vi "Exit.vi"(8 "error in (no error)":errorcluster, 11 "Running in":refnum<class "Running.lvclass">) -> (0 "error out":errorcluster, 3 "Running out":refnum<class "Running.lvclass">)   [LabVIEW 2013, in "Process States.lvlib" / "Running.lvclass"]
doc: "This override sends a Stop Acquisition message to the Process Actor. It also sends a Log Event message to the UI, with the string containing \"Exiting Running State\", the average value of the data stream, and the total number of elements of the steam as its payload."
uses:
  Running.lvclass
  <vilib>/ActorFramework/Actor/Actor.lvclass/Actor.ctl
  Process State/Process State.lvclass
  Process State/Process State.lvclass/Process State.ctl
  Running.lvclass/Running.ctl
  State Pattern UI/Log Event Msg/Log Event Msg.lvclass/Log Event Msg.ctl
  <vilib>/ActorFramework/Message Enqueuer/Message Enqueuer.lvclass/Message Enqueuer.ctl
  <vilib>/ActorFramework/Message Enqueuer/Enqueue.vi
  <vilib>/ActorFramework/Message Priority Queue/Priority Enqueue.vi
  State Pattern UI/Log Event Msg/Log Event Msg.lvclass
  Process Actor/Process Messages/Stop Acquisition Msg/Stop Acquisition Msg.lvclass
  <vilib>/ActorFramework/Actor/Actor.lvclass
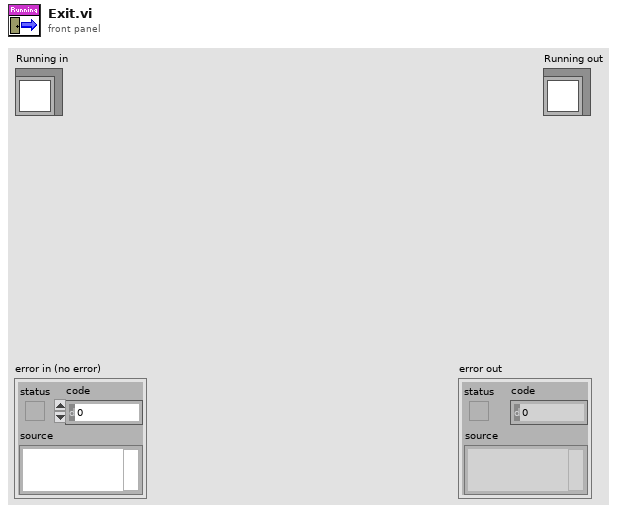
[diagram p1: front panel]
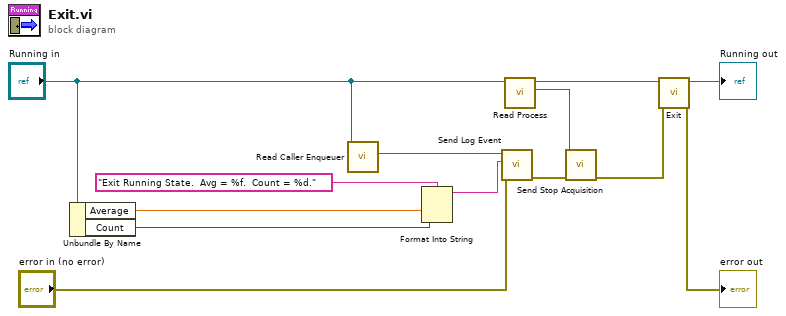
[diagram p0: block diagram]
diagram:
  n1 = Unbundle By Name("Running in") -> ("Average"=w13:dbl, "Count"=w10:i32)
  n2 = call <vilib>:"Read Caller Enqueuer.vi"("Actor"="Running in") -> ("Caller Enqueuer"=w9:refnum<class "Message Enqueuer.lvclass">)  [unwired: 10 in]
  n3 = Format Into String(format string="Exit Running State.  Avg = %f.  Count = %d." ("Event Text"), w13, w10) -> (resulting string=w11:string)  [unwired: 2 in, 1 out]
  n4 = call "Send Log Event.vi"("error in (no error)"="error in (no error)", "Event Text"=w11, "Message Enqueuer"=w9) -> ("error out"=w4:errorcluster)  [unwired: 8 in]
  n5 = call "Read Process.vi"("Process State in"="Running in") -> ("Process Enqueuer"=w5:refnum<class "Message Enqueuer.lvclass">, "Process State out"=w6:refnum<class "Running.lvclass">)  [unwired: 9 in]
  n6 = call "Send Stop Acquisition.vi"("error in (no error)"=w4, "Message Enqueuer"=w5) -> ("error out"=w2:errorcluster)  [unwired: 8 in, 1 out]
  n7 = call-parent "Exit.vi"("error in (no error)"=w2, "Old State"=w6) -> ("error out"=→"error out":errorcluster, "New State"=→"Running out":refnum<class "Running.lvclass">)  [unwired: 8 in]
